vi "Get Element Read Position.vi"(8 "error in (no error)":errorcluster, 11 "CIPC Reference":u64) -> (0 "error out":errorcluster, 3 "Element Read Position":u32)   [LabVIEW 2021, in "CIF_NI_CIPC.lvlib"]
doc: "Get element position in the CIPC buffer from which the next element will be read."
uses:
  CIF_NI_CIPC.lvlib
  <vilib>/Utility/error.llb/Trim Whitespace.vi
  <vilib>/Utility/error.llb/Error Cluster From Error Code.vi
  libnicipc.dll
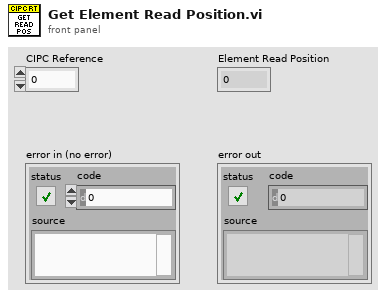
[diagram p1: front panel]
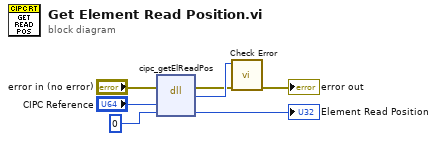
[diagram p0: block diagram]
diagram:
  n1 = dll-call lib="libnicipc.*" fn="cipc_getElReadPos"(error in="error in (no error)", "cipc_buffer_ref"="CIPC Reference", "el_index"=u32 0) -> (error out=w3:errorcluster, "return type"=w4:i32, "el_index"=→"Element Read Position":u32)  [unwired: 3 in, 1 out]
  n2 = call "Check Error.vi"("error in (no error)"=w3, "Error Code"=w4) -> ("error out"=→"error out":errorcluster)  [unwired: 9 in]
